vi "Write Handle Injections.vi"(8 "error in (no error)":errorcluster, 10 "Handle Injections":bool, 11 "InteractionProcessor in":refnum<class "InteractionProcessor.lvclass">) -> (0 "error out":errorcluster, 3 "InteractionProcessor out":refnum<class "InteractionProcessor.lvclass">)   [LabVIEW 2023, in "HAF.lvlib" / "InteractionProcessor.lvclass"]
uses:
  InteractionProcessor.lvclass
  InteractionProcessor.lvclass/InteractionProcessor.ctl
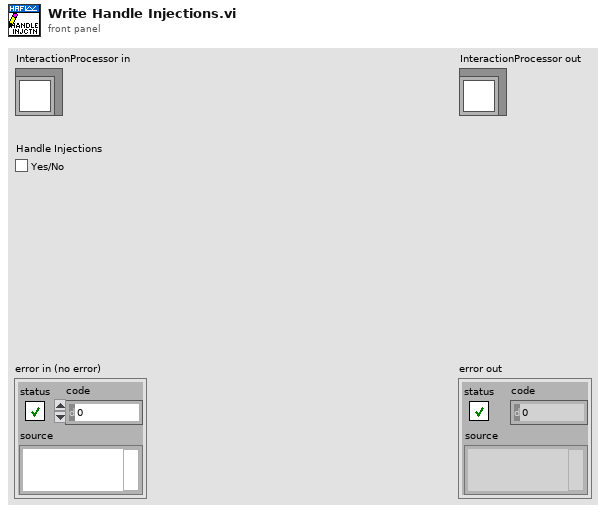
[diagram p1: front panel]
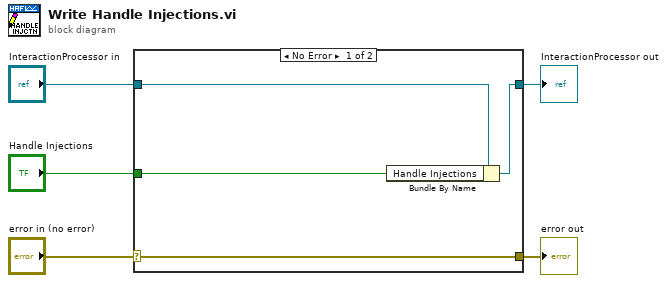
[diagram p0: block diagram]
diagram:
  n1 = case shown="No Error" "error in (no error)" {
    selector: "error in (no error)" -> [w9 w10]
    tunnel: [w9 w10] -> w4
    tunnel: [w7 w11] -> w2
    tunnel: "InteractionProcessor in" -> [w8 w11]
    tunnel: "Handle Injections" -> [w6 _]
    frame No Error {
      n2 = Bundle By Name(cluster=w8, "Handle Injections"=w6) -> (w7:refnum<class "InteractionProcessor.lvclass">)
    }
    frame Error {
    }
  }
  "error out" <- w4
  "InteractionProcessor out" <- w2
